vi "P541_scanning.vi"(6 "Velocity":dbl, 8 "Axis":bool[](array[boolean]), 9 "Positions":dbl[](array[numeric]), 10 "Action":T1, 11 "VISA resource name":refnum<visa-resource-name>) -> (0 "Special Function":string, 1 "Status":bool, 2 "Position Out":dbl[](array[numeric]))   [LabVIEW 2011]
uses:
  Controls/StageStates.ctl
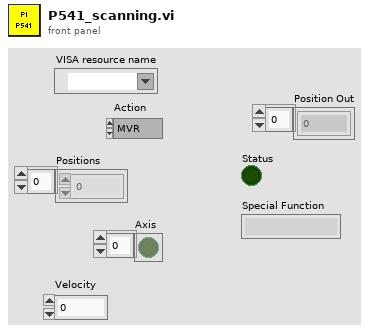
[diagram p1: front panel]
types:
  T1 = typedef "StageStates.ctl" = enum16{"MVR", "MOVE", "HALT", "ONTARGET", "ERROR", "EXIT", "HOME", "ZEROPOS", "NANOPOS", "QUIT", "ANALOG"}
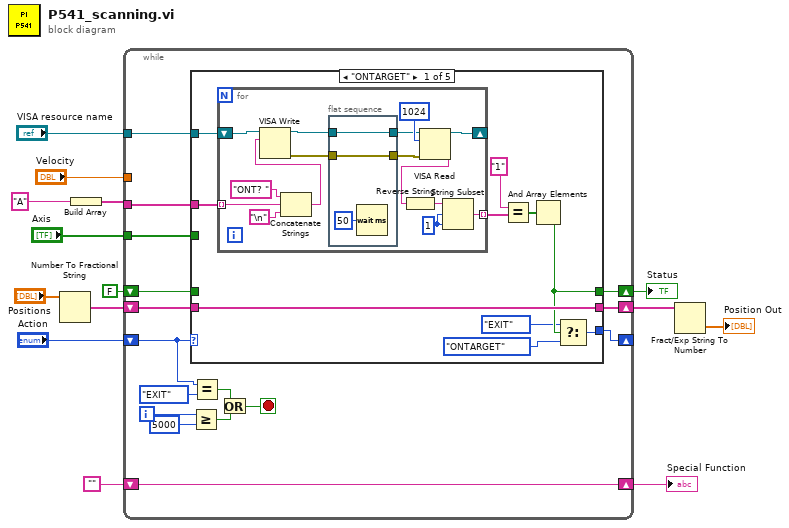
[diagram p0: block diagram]
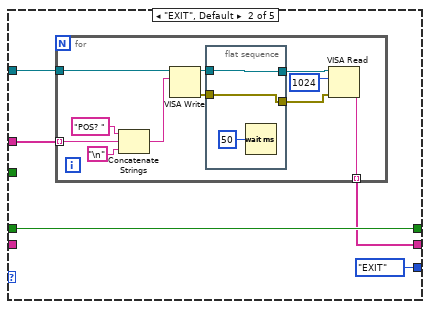
[diagram p2: hidden frame]
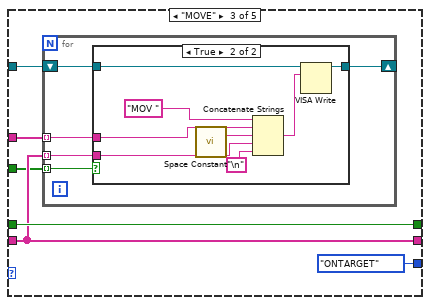
[diagram p3: hidden frame]
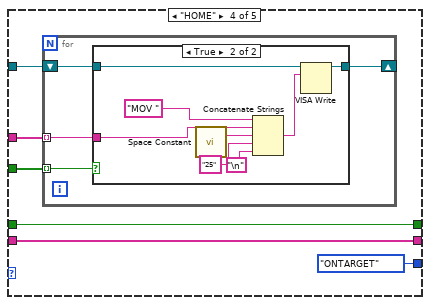
[diagram p5: hidden frame]
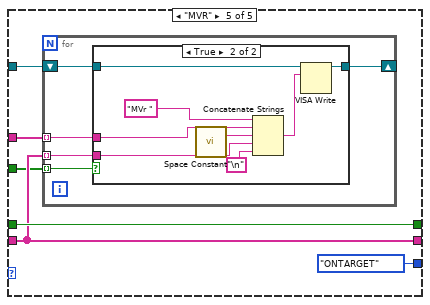
[diagram p7: hidden frame]
diagram:
  n1 = Number To Fractional String(number="Positions") -> (F-format string=w4:string[])  [unwired: 3 in]
  n2 = Build Array("A") -> (w9:string[])
  n3 = while {
    tunnel: w9 -> [w30]
    tunnel: "VISA resource name" -> [w29]
    shift-right: [w15] -> _
    shift-left: "Action" -> [w24]
    shift-right: [w27] -> w3
    shift-left: w4 -> [w28]
    shift-right: [w25] -> w12
    shift-left: FALSE -> [w26]
    tunnel: "Axis" -> [w18]
    shift-right: [w16] -> w6
    shift-left: "" -> [w16]
    tunnel: "Velocity" -> [_]
    i -> [w22]
    stop <- w20 stop-if-true
    n4 = case shown="\"ONTARGET\"" w24 {
      tunnel: w30 -> [w40 w63 w83 w103 w122]
      tunnel: w29 -> [w34 w61 w82 w102 w121]
      tunnel: w28 -> [w36 _ w80 w100 w119]
      tunnel: [w36 w60 w80 w100 w119] -> w27
      tunnel: w26 -> [_ w62 w81 w101 w120]
      tunnel: [w35 w62 w81 w101 w120] -> w25
      tunnel: w18 -> [_ _ w79 w99 w118]
      tunnel: [w31 StageStates."EXIT" ("Action") StageStates."ONTARGET" ("Action") StageStates."ONTARGET" ("Action") StageStates."ONTARGET" ("Action")] -> w15
      frame "ONTARGET" {
        n5 = for {
          tunnel: w40 -> [w55] mode=indexing
          tunnel: [w54] -> w39 mode=indexing
          shift-right: [w45] -> _
          shift-left: w34 -> [w46]
          w49 = 1 ("length (rest)")
          n6 = Concatenate Strings("ONT? " ("string"), w55, "\n") -> (w48:string)
          n7 = VISA Write(VISA resource name=w46, write buffer=w48) -> (VISA resource name out=w43:refnum<visa-resource-name>, error out=w41:errorcluster)  [unwired: 1 in, 1 out]
          n8 = flat-sequence {
            tunnel: [w58] -> w44
            tunnel: w43 -> [w58]
            tunnel: [w57] -> w42
            tunnel: w41 -> [w57]
            frame #0 {
              n9 = Wait (ms)(milliseconds to wait=u32 50) -> ()  [unwired: 1 out]
            }
          }
          n10 = VISA Read(VISA resource name=w44, byte count=u32 1024, error in (no error)=w42) -> (VISA resource name out=w45:refnum<visa-resource-name>, read buffer=w47:string)  [unwired: 2 out]
          n11 = Reverse String(1:w47) -> (0:w50:string)
          n12 = String Subset(string=w50, offset (0)=w49, length (rest)=w49) -> (substring=w54:string)
        }
        n13 = Equal?(x="1", y=w39) -> (x = y?=w37:bool[])
        n14 = And Array Elements(Boolean array=w37) -> (logical AND=w35:bool)
        n15 = Select(t=StageStates."EXIT" ("Action"), s=w35, f=StageStates."ONTARGET" ("Action")) -> (s? t:f=w31:T1)
      }
      frame "EXIT", Default {
        n16 = for {
          tunnel: w63 -> [w74] mode=indexing
          tunnel: w61 -> [w69]
          tunnel: [w68] -> w60 mode=indexing
          n17 = Concatenate Strings("POS? " ("string"), w74, "\n") -> (w70:string)
          n18 = VISA Write(VISA resource name=w69, write buffer=w70) -> (VISA resource name out=w66:refnum<visa-resource-name>, error out=w64:errorcluster)  [unwired: 1 in, 1 out]
          n19 = flat-sequence {
            tunnel: [w77] -> w67
            tunnel: w66 -> [w77]
            tunnel: [w76] -> w65
            tunnel: w64 -> [w76]
            frame #0 {
              n20 = Wait (ms)(milliseconds to wait=u32 50) -> ()  [unwired: 1 out]
            }
          }
          n21 = VISA Read(VISA resource name=w67, byte count=u32 1024, error in (no error)=w65) -> (read buffer=w68:string)  [unwired: 3 out]
        }
      }
      frame "MOVE" {
        n22 = for {
          tunnel: w83 -> [w88] mode=indexing
          tunnel: w80 -> [w87] mode=indexing
          shift-right: [w85] -> _
          shift-left: w82 -> [w86]
          tunnel: w79 -> [w84] mode=indexing
          n23 = case shown="True" w84 {
            tunnel: w88 -> [_ w95]
            tunnel: w87 -> [_ w92]
            tunnel: w86 -> [w89 w91]
            tunnel: [w89 w90] -> w85
            frame False {
            }
            frame True {
              n24 = call <vilib>:"Space Constant.vi"() -> ("String"=w93:string)
              n25 = Concatenate Strings("MOV ", w95, w93, w92, "\n") -> (w97:string)
              n26 = VISA Write(VISA resource name=w91, write buffer=w97) -> (VISA resource name out=w90:refnum<visa-resource-name>)  [unwired: 1 in, 2 out]
            }
          }
        }
      }
      frame "HOME" {
        n27 = for {
          tunnel: w103 -> [w107] mode=indexing
          shift-right: [w105] -> _
          shift-left: w102 -> [w106]
          tunnel: w99 -> [w104] mode=indexing
          n28 = case shown="True" w104 {
            tunnel: w107 -> [_ w114]
            tunnel: w106 -> [w108 w111]
            tunnel: [w108 w110] -> w105
            frame False {
            }
            frame True {
              n29 = call <vilib>:"Space Constant.vi"() -> ("String"=w112:string)
              n30 = Concatenate Strings("MOV ", w114, w112, "25" ("string"), "\n") -> (w116:string)
              n31 = VISA Write(VISA resource name=w111, write buffer=w116) -> (VISA resource name out=w110:refnum<visa-resource-name>)  [unwired: 1 in, 2 out]
            }
          }
        }
      }
      frame "MVR" {
        n32 = for {
          tunnel: w122 -> [w127] mode=indexing
          tunnel: w119 -> [w126] mode=indexing
          shift-right: [w124] -> _
          shift-left: w121 -> [w125]
          tunnel: w118 -> [w123] mode=indexing
          n33 = case shown="True" w123 {
            tunnel: w127 -> [_ w134]
            tunnel: w126 -> [_ w131]
            tunnel: w125 -> [w128 w130]
            tunnel: [w128 w129] -> w124
            frame False {
            }
            frame True {
              n34 = call <vilib>:"Space Constant.vi"() -> ("String"=w132:string)
              n35 = Concatenate Strings("MVr ", w134, w132, w131, "\n") -> (w136:string)
              n36 = VISA Write(VISA resource name=w130, write buffer=w136) -> (VISA resource name out=w129:refnum<visa-resource-name>)  [unwired: 1 in, 2 out]
            }
          }
        }
      }
    }
    n37 = Greater Or Equal?(x=w22, y=5000) -> (x >= y?=w19:bool)
    n38 = Equal?(x=w24, y=StageStates."EXIT") -> (x = y?=w23:bool)
    n39 = Or(x=w23, y=w19) -> (x .or. y?=w20:bool)
  }
  "Status" <- w12
  "Special Function" <- w6
  n40 = Fract/Exp String To Number(string=w3) -> (number=→"Position Out":dbl[])  [unwired: 3 in, 1 out]
